vi "Get Signal Names.vi"(8 "error in (no error)":errorcluster, 11 "Module in":refnum<class "Module.lvclass">) -> (0 "error out":errorcluster, 2 "Signal Names":string[](array[string]), 3 "Module out":refnum<class "Module.lvclass">)   [LabVIEW 2015, in "Module.lvclass"]
uses:
  Module.lvclass
  Module.lvclass/Module.ctl
  IO/IO Class/IO Class.lvclass
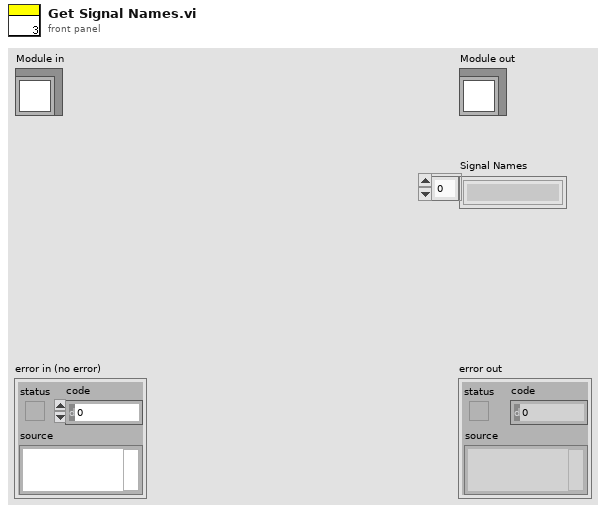
[diagram p1: front panel]
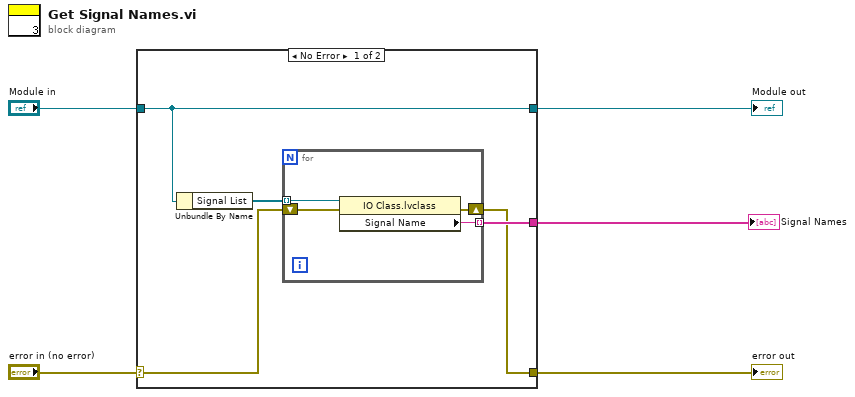
[diagram p0: block diagram]
diagram:
  n1 = case shown="No Error" "error in (no error)" {
    selector: "error in (no error)" -> [w7 w16]
    tunnel: [w6 w16] -> w3
    tunnel: [w10 w15] -> w1
    tunnel: "Module in" -> [w10 w15]
    tunnel: [w8 _] -> w2
    frame No Error {
      n2 = Unbundle By Name(w10) -> ("Signal List"=w9:refnum<class "IO Class.lvclass">[])
      n3 = for {
        tunnel: w9 -> [w14] mode=indexing
        tunnel: [w13] -> w8 mode=indexing
        shift-right: [w11] -> w6
        shift-left: w7 -> [w12]
        n4 = property class="IO Class.lvclass"(reference=w14, error in=w12) -> (error out=w11:errorcluster, "Signal Name"=w13:string)  [unwired: 1 out]
      }
    }
    frame Error {
    }
  }
  "error out" <- w3
  "Module out" <- w1
  "Signal Names" <- w2
